vi "Paralell Vectors XY.vi"(10 "Vector 2":i64[](array[numeric]), 11 "Vector 1":i64[](array[numeric])) -> (3 "Boolean":bool)   [LabVIEW 2021, in "Vector.lvclass"]
uses:
  Vector.lvclass
  Vector.lvclass/Vector.ctl
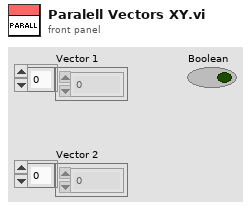
[diagram p1: front panel]
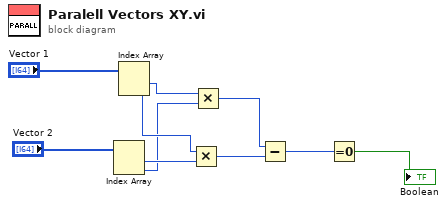
[diagram p0: block diagram]
diagram:
  n1 = Index Array(array="Vector 2") -> (element #1=w6:i64, element #2=w4:i64)  [unwired: 2 in]
  n2 = Index Array(array="Vector 1") -> (element #1=w3:i64, element #2=w5:i64)  [unwired: 2 in]
  n3 = Multiply(x=w5, y=w6) -> (x*y=w8:i64)
  n4 = Multiply(x=w3, y=w4) -> (x*y=w7:i64)
  n5 = Subtract(x=w7, y=w8) -> (x-y=w9:i64)
  n6 = Equal To 0?(x=w9) -> (x = 0?=→"Boolean":bool)
